vi "ConfigureVirtualChannelModule.vi"(8 "error in (no error)":errorcluster) -> (0 "error out":errorcluster, 1 "register data sets":T1[](array[typedef]), 3 "Virtual Channel Config":T4)   [LabVIEW 2017, in "CmsVirtualChannel.lvlib"]
uses:
  <vilib>/addons/InsightCM/Devices/Shared/Cms/CmsVirtualChannel/CmsVirtualChannel.lvlib
  <vilib>/addons/InsightCM/Devices/Shared/Cms/CmsVirtualChannel/controls/Config.ctl
  <vilib>/addons/InsightCM/Devices/Shared/Cms/CmsVirtualChannel/controls/VirtualChannelGroup.ctl
  <vilib>/addons/InsightCM/Devices/Shared/Cms/CmsVirtualChannel/controls/VirtualChannel.ctl
  <vilib>/addons/InsightCM/Devices/Shared/Common/DataEventCreator/controls/RegisterDataSets.ctl
  <vilib>/addons/InsightCM/Devices/Shared/Cms/CmsDataEventCreator/controls/DataSetRegistry.ctl
  <vilib>/addons/InsightCM/Devices/Shared/Common/DataEvent/controls/DataSetType.ctl
  <vilib>/addons/InsightCM/MessageBus/Base/controls/R2_DeviceModel.ctl
  <vilib>/addons/InsightCM/MessageBus/Base/controls/R2_Device.ctl
  <vilib>/addons/InsightCM/MessageBus/Base/controls/KeyValuePair.ctl
  <vilib>/addons/InsightCM/MessageBus/Base/controls/DeviceState.ctl
  <vilib>/addons/InsightCM/MessageBus/Base/controls/R2_DataGroup.ctl
  <vilib>/addons/InsightCM/MessageBus/Base/controls/OperatingState.ctl
  <vilib>/addons/InsightCM/MessageBus/Base/controls/Trigger.ctl
  <vilib>/addons/InsightCM/MessageBus/Base/controls/Condition.ctl
  <vilib>/addons/InsightCM/MessageBus/Base/controls/BurstModeTrigger.ctl
  <vilib>/addons/InsightCM/MessageBus/Base/controls/R2_Channel.ctl
  <vilib>/addons/InsightCM/MessageBus/Base/controls/Metric.ctl
  <vilib>/addons/InsightCM/MessageBus/Base/controls/Tag.ctl
  <vilib>/addons/InsightCM/Utilities/GlobalConfiguration/GlobalConfiguration.lvlib
  <vilib>/addons/InsightCM/Utilities/DeviceModelHelpers/DeviceModelHelpers.lvlib
  <vilib>/addons/InsightCM/Utilities/PropertyHelpers/PropertyHelpers.lvlib
  <vilib>/addons/InsightCM/Devices/Shared/Cms/CmsAcquisition/CmsAcquisition.lvlib
  <vilib>/addons/InsightCM/Devices/Shared/Common/DataEvent/DataEvent.lvlib
  <vilib>/addons/InsightCM/Devices/Shared/Cms/CmsDataEventCreator/CmsDataEventCreator.lvlib
  <vilib>/addons/InsightCM/Devices/Shared/Common/DataEventCreator/DataEventCreator.lvlib
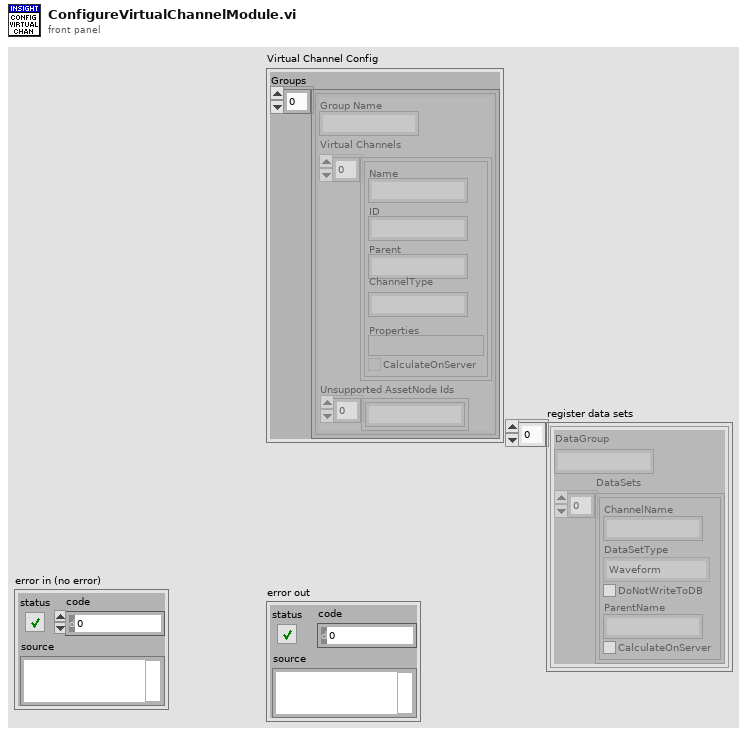
[diagram p1: front panel]
types:
  T1 = typedef "DataEventCreator.lvlib/RegisterDataSets.ctl" = cluster{"DataGroup":string, "DataSets":T2[]}
  T2 = typedef "CmsDataEventCreator.lvlib/DataSetRegistry.ctl" = cluster{"ChannelName":string, "DataSetType":T3, "DoNotWriteToDB":bool, "ParentName":string, "CalculateOnServer":bool}
  T3 = typedef "DataEvent.lvlib/DataSetType.ctl" = enum16{"Waveform", "SpeedProfile", "ThermalImage", "EmsaSweep"}
  T4 = typedef "CmsVirtualChannel.lvlib/Config.ctl" = cluster{"Groups":T5[]}
  T5 = typedef "CmsVirtualChannel.lvlib/VirtualChannelGroup.ctl" = cluster{"Group Name":string, "Virtual Channels":T6[], "Unsupported AssetNode Ids":string[]}
  T6 = typedef "CmsVirtualChannel.lvlib/VirtualChannel.ctl" = cluster{"Name":string, "ID":string, "Parent":string, "ChannelType":string, "Properties":variant, "CalculateOnServer":bool}
  T7 = typedef "R2_DeviceModel.ctl" = cluster{"Device":T8, "Channels":T16[], "Tags":T18[]}
  T8 = typedef "R2_Device.ctl" = cluster{"Id":string, "Name":string, "DeviceType":string, "HardwareName":string, "IpAddress":string, "HardwareInfo":T9[], "ApplicationType":string, "ApplicationVersion":string, "EquipmentIds":string[], "ConfigurationVersion":string, "State":T10, "Properties":T9[], "DataGroups":T11[], "BurstModeTrigger":T15}
  T9 = typedef "KeyValuePair.ctl" = cluster{"Key":string, "Value":string}
  T10 = typedef "DeviceState.ctl" = cluster{"Disabled":bool}
  T11 = typedef "R2_DataGroup.ctl" = cluster{"Name":string, "OperatingStates":T12[], "Properties":T9[], "EquipmentIds":string[], "AssetNodeId":string}
  T12 = typedef "OperatingState.ctl" = cluster{"Name":string, "Properties":T9[], "Triggers":T13[]}
  T13 = typedef "Trigger.ctl" = cluster{"Type":string, "Expression":string, "Conditions":T14[]}
  T14 = typedef "Condition.ctl" = cluster{"Source":string, "Type":string, "Operator":string, "CompareTo":string, "DwellSeconds":dbl}
  T15 = typedef "BurstModeTrigger.ctl" = cluster{"Trigger":T13, "SampleRate":string, "AcquisitionLength":string}
  T16 = typedef "R2_Channel.ctl" = cluster{"Id":string, "DeviceId":string, "Name":string, "ChannelType":string, "HardwareKey":string, "HardwareChannel":string, "DataGroup":string, "Keywords":string[], "EquipmentIds":string[], "Properties":T9[], "Metrics":T17[], "AssetNodeId":string, "MeasType":string, "AssetName":string}
  T17 = typedef "Metric.ctl" = cluster{"Id":string, "Name":string, "Unit":string, "Properties":T9[], "MetricDefinitionInstanceId":string}
  T18 = typedef "Tag.ctl" = cluster{"Id":string, "Path":string, "Name":string, "Datatype":string, "Props":T9[], "Keywords":string[]}
  T19 = typedef "SectionKeyValues.ctl" = cluster{"Section":string, "KeyValues":T9[]}
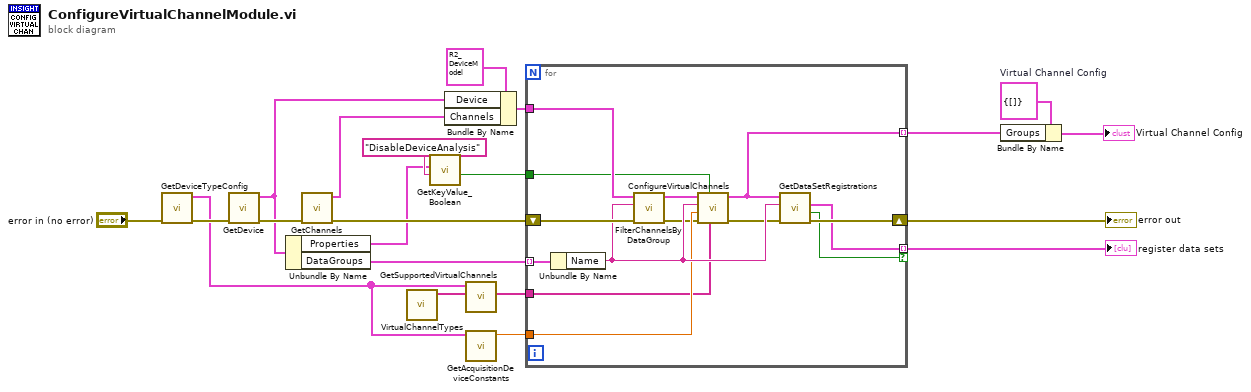
[diagram p0: block diagram]
diagram:
  w16 = T4 {"Groups"=[]}  # Virtual Channel Config
  n1 = call <vilib>:"GetDeviceTypeConfig.vi"("error in (no error)"="error in (no error)") -> ("error out"=w5:errorcluster, "key values"=w4:T19[])  [unwired: 8 in, 1 out]
  n2 = call <vilib>:"GetDevice.vi"("error in (no error)"=w5) -> ("error out"=w21:errorcluster, "device configuration"=w14:T8)  [unwired: 8 in, 1 out]
  n3 = Unbundle By Name(w14) -> ("Properties"=w8:T9[], "DataGroups"=w20:T11[])
  n4 = call <vilib>:"GetChannels.vi"("error in (no error)"=w21) -> ("error out"=w18:errorcluster, "channels"=w13:T16[])  [unwired: 8 in, 1 out]
  n5 = call <vilib>:"VirtualChannelTypes.vi"() -> ("Array"=w1:string[])  [unwired: 11 in]
  n6 = call <vilib>:"GetKeyValue_Boolean.vi"("key"="DisableDeviceAnalysis", "key value pairs"=w8) -> ("value"=w7:bool)  [unwired: 7 in, 2 out]
  n7 = Bundle By Name(cluster=T7 {"Device"={"Id"="", "Name"="", "DeviceType"="", "HardwareName"="", "IpAddress"="", "HardwareInfo"=[], "ApplicationType"="", "ApplicationVersion"="", "EquipmentIds"=[], "ConfigurationVersion"="", "State"={"Disabled"=FALSE}, "Properties"=[], "DataGroups"=[], "BurstModeTrigger"={"Trigger"={"Type"="", "Expression"="", "Conditions"=[]}, "SampleRate"="", "AcquisitionLength"=""}}, "Channels"=[], "Tags"=[]} ("device model"), "Device"=w14, "Channels"=w13) -> (w12:T7)
  n8 = call <vilib>:"GetSupportedVirtualChannels.vi"("default virtual channel types"=w1, "key values"=w4) -> ("not supported virtual channels"=w10:string[])  [unwired: 9 in]
  n9 = call <vilib>:"GetAcquisitionDeviceConstants.vi"("key values"=w4) -> ("settling time (seconds)"=w3:dbl)  [unwired: 10 in]
  n10 = for {
    shift-right: [w35] -> w19
    shift-left: w18 -> [w30]
    tunnel: w20 -> [w31] mode=indexing
    tunnel: [w34] -> w6 mode=indexing if=w33
    tunnel: w12 -> [w32]
    tunnel: w10 -> [w23]
    tunnel: w7 -> [w28]
    tunnel: w3 -> [w26]
    tunnel: [w22] -> w2 mode=indexing
    n11 = Unbundle By Name(w31) -> ("Name"=w29:string)
    n12 = call <vilib>:"FilterChannelsByDataGroup.vi"("error in (no error)"=w30, "group"=w29, "device model"=w32) -> ("error out"=w24:errorcluster, "channels in data group"=w25:T16[])  [unwired: 7 in]
    n13 = call <vilib>:"ConfigureVirtualChannels.vi"("not supported virtual channels"=w23, "DisableDeviceAnalysis"=w28, "error in (no error)"=w24, "settling time (seconds)"=w26, "data group name"=w29, "channels in this group"=w25) -> ("error out"=w27:errorcluster, "virtual channel config"=w22:T5)  [unwired: 3 in, 1 out]
    n14 = call <vilib>:"GetDataSetRegistrations.vi"("error in (no error)"=w27, "data group name"=w29, "virtual channel config"=w22) -> ("error out"=w35:errorcluster, "atleast one data set to register"=w33:bool, "register data set"=w34:T1)  [unwired: 6 in]
  }
  "error out" <- w19
  "register data sets" <- w6
  n15 = Bundle By Name(cluster=w16, "Groups"=w2) -> (→"Virtual Channel Config":T4)
